vi "Latihan 12 (Control Kecepatan).vi"() -> ()   [LabVIEW 2021]
panel:
  in  "stop":bool
  in  "Nama":string
  in  "Password":string
  in  "Login":bool
  in  "KECEPATAN":dbl(knob) scale=1.0..10.0
  in  "Tab Control 2":enum32{"Page 1", "Page 2", "Page 3"}(tab)
  in  "Tab Control":enum32{"Page 1", "Page 2", "Page 3"}(tab)
  # "KEPADA"
  # "TAMU UNDANGAN"
  # "SURAKARTA"
  # "TERIMA KASIH"
  # "YANG TERHORMAT"
  # "POLITEKNIK ATMI"
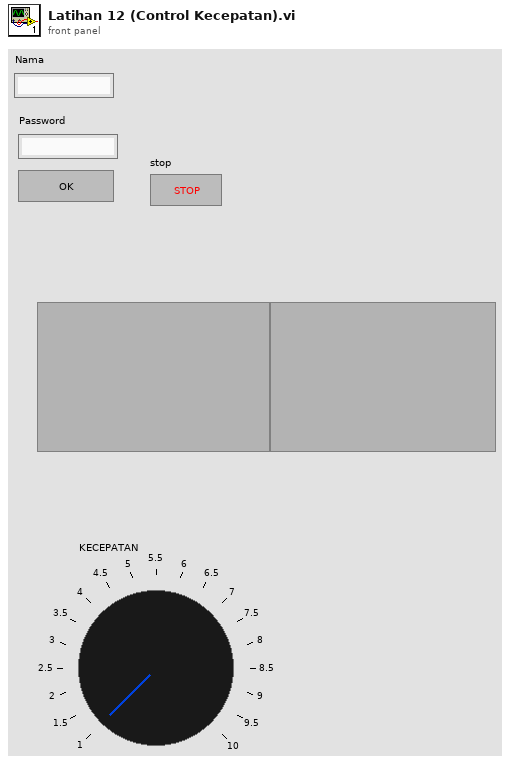
[diagram p1: front panel]
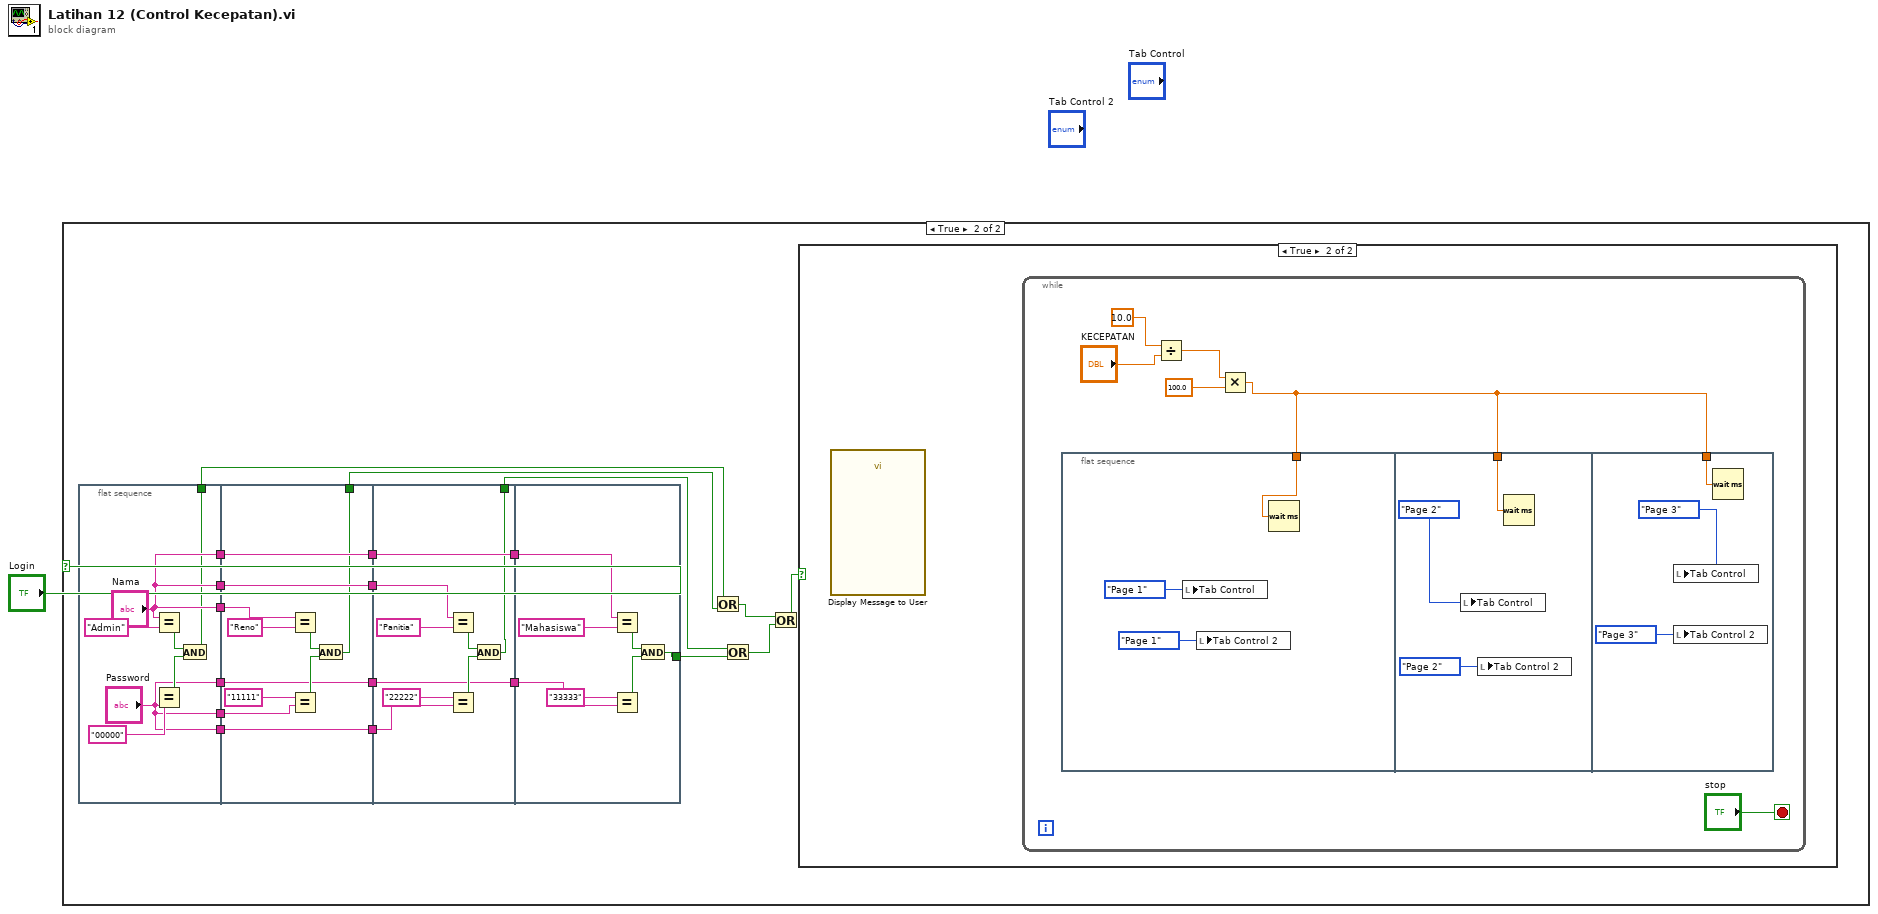
[diagram p0: block diagram]
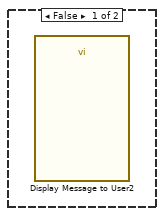
[diagram p3: hidden frame]
diagram:
  n1 = case shown="True" "Login" {
    frame False {
    }
    frame True {
      n2 = flat-sequence {
        tunnel: ["Nama"] -> w20
        tunnel: ["Nama"] -> w18
        tunnel: ["Nama"] -> w15
        tunnel: ["Password"] -> w14
        tunnel: ["Password"] -> w12
        tunnel: ["Password"] -> w9
        tunnel: [w21] -> w2
        tunnel: w20 -> [w36]
        tunnel: [w35] -> w19
        tunnel: w18 -> [w35]
        tunnel: [w34] -> w16
        tunnel: w15 -> [w34]
        tunnel: w14 -> [w33]
        tunnel: [w32] -> w13
        tunnel: w12 -> [w32]
        tunnel: [w31] -> w10
        tunnel: w9 -> [w31]
        tunnel: [w28] -> w3
        tunnel: w19 -> [w45]
        tunnel: [w44] -> w17
        tunnel: w16 -> [w44]
        tunnel: w13 -> [w43]
        tunnel: [w42] -> w11
        tunnel: w10 -> [w42]
        tunnel: [w39] -> w4
        tunnel: w17 -> [w52]
        tunnel: w11 -> [w51]
        tunnel: [w48] -> w5
        frame #0 {
          n3 = Equal?(x="Nama", y="Admin") -> (x = y?=w25:bool)
          n4 = Equal?(x="00000", y="Password") -> (x = y?=w24:bool)
          n5 = And(x=w25, y=w24) -> (x .and. y?=w21:bool)
        }
        frame #1 {
          n6 = Equal?(x=w36, y="Reno") -> (x = y?=w38:bool)
          n7 = Equal?(x="11111", y=w33) -> (x = y?=w37:bool)
          n8 = And(x=w38, y=w37) -> (x .and. y?=w28:bool)
        }
        frame #2 {
          n9 = Equal?(x=w45, y="Panitia") -> (x = y?=w47:bool)
          n10 = Equal?(x="22222", y=w43) -> (x = y?=w46:bool)
          n11 = And(x=w47, y=w46) -> (x .and. y?=w39:bool)
        }
        frame #3 {
          n12 = Equal?(x=w52, y="Mahasiswa") -> (x = y?=w54:bool)
          n13 = Equal?(x="33333", y=w51) -> (x = y?=w53:bool)
          n14 = And(x=w54, y=w53) -> (x .and. y?=w48:bool)
        }
      }
      n15 = Or(x=w2, y=w3) -> (x .or. y?=w8:bool)
      n16 = Or(x=w4, y=w5) -> (x .or. y?=w7:bool)
      n17 = Or(x=w8, y=w7) -> (x .or. y?=w6:bool)
      n18 = case shown="True" w6 {
        frame False {
          n19 = call "Display Message to User2"() -> ()  [unwired: 10 in, 2 out]
        }
        frame True {
          n20 = call "Display Message to User"() -> ()  [unwired: 10 in, 2 out]
          n21 = while {
            stop <- "stop" stop-if-true
            n22 = flat-sequence {
              tunnel: w59 -> [w61]
              tunnel: w59 -> [w64]
              tunnel: w59 -> [w67]
              frame #0 {
                n23 = local write "Tab Control"(enum32{"Page 1", "Page 2", "Page 3"}."Page 1" ("Tab Control")) -> ()
                n24 = local write "Tab Control 2"(enum32{"Page 1", "Page 2", "Page 3"}."Page 1" ("Tab Control 2")) -> ()
                n25 = Wait (ms)(milliseconds to wait=w61) -> ()  [unwired: 1 out]
              }
              frame #1 {
                n26 = local write "Tab Control"(enum32{"Page 1", "Page 2", "Page 3"}."Page 2" ("Tab Control")) -> ()
                n27 = local write "Tab Control 2"(enum32{"Page 1", "Page 2", "Page 3"}."Page 2" ("Tab Control 2")) -> ()
                n28 = Wait (ms)(milliseconds to wait=w64) -> ()  [unwired: 1 out]
              }
              frame #2 {
                n29 = local write "Tab Control"(enum32{"Page 1", "Page 2", "Page 3"}."Page 3" ("Tab Control")) -> ()
                n30 = local write "Tab Control 2"(enum32{"Page 1", "Page 2", "Page 3"}."Page 3" ("Tab Control 2")) -> ()
                n31 = Wait (ms)(milliseconds to wait=w67) -> ()  [unwired: 1 out]
              }
            }
            n32 = Divide(x=10.0, y="KECEPATAN") -> (x/y=w56:dbl)
            n33 = Multiply(x=w56, y=100.0) -> (x*y=w59:dbl)
          }
        }
      }
    }
  }
